vi "Create Task.vi"(8 "error in":errorcluster, 10 "Task name":string="AnalogInputTask", 11 "Analog Input in":refnum<class "NI Analog Input.lvclass">) -> (0 "error out":errorcluster, 3 "Analog Input out":refnum<class "NI Analog Input.lvclass">)   [LabVIEW 2023, in "HardwareAbstractionLayer_LVOOP.lvlib" / "NI Analog Input.lvclass"]
doc: "This VI Device Create Task"
uses:
  NI Analog Input.lvclass
  NI Analog Input.lvclass/NI Analog Input.ctl
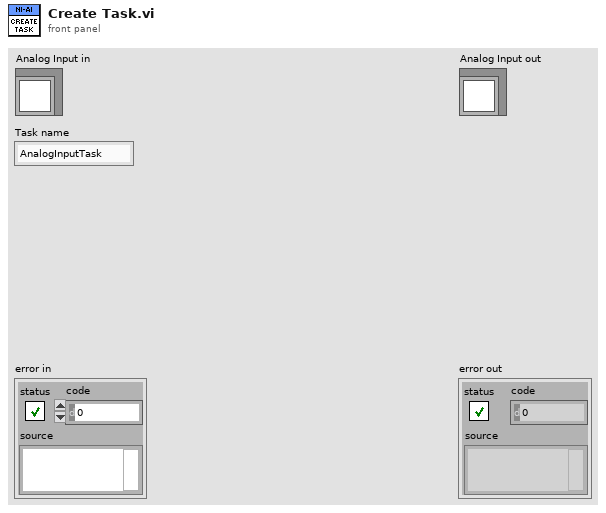
[diagram p1: front panel]
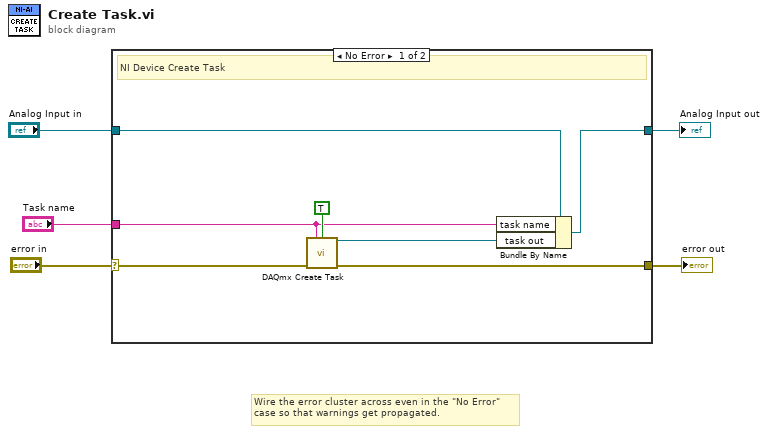
[diagram p0: block diagram]
diagram:
  # "Wire the error cluster across even in the \"No Error\"\ncase so that warnings get propagated."
  n1 = case shown="No Error" "error in" {
    selector: "error in" -> [w12 w14]
    tunnel: [w11 w14] -> w4
    tunnel: [w9 w13] -> w2
    tunnel: "Analog Input in" -> [w10 w13]
    tunnel: "Task name" -> [w6 _]
    frame No Error {
      # "NI Device Create Task"
      n2 = call <vilib>:"DAQmx Create Task.vi"("new task name"=w6, "auto cleanup"=TRUE, "error in"=w12) -> ("task out"=w8:refnum<k21>, "error out"=w11:errorcluster)  [unwired: 11 in]
      n3 = Bundle By Name(cluster=w10, "task name"=w6, "task out"=w8) -> (w9:refnum<class "NI Analog Input.lvclass">)
    }
    frame Error {
    }
  }
  "error out" <- w4
  "Analog Input out" <- w2
